vi "medidorIXV.vi"() -> (2 "Corrente Atual":dbl, 3 "Tensao Atual":dbl)   [LabVIEW 2012]
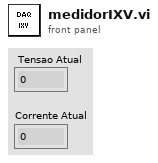
[diagram p1: front panel]
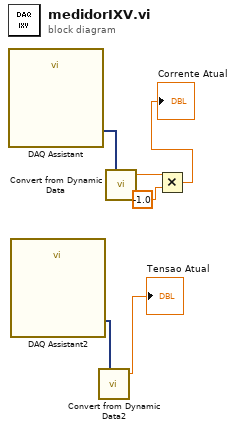
[diagram p0: block diagram]
diagram:
  n1 = call "DAQ Assistant"() -> ("data"=w3:dynamicdata)  [unwired: 17 in, 2 out]
  n2 = call "DAQ Assistant2"() -> ("data"=w1:dynamicdata)  [unwired: 17 in, 2 out]
  n3 = call "Convert from Dynamic Data2"("Dynamic Data Type"=w1) -> ("Scalar"=→"Tensao Atual":dbl)  [unwired: 3 in]
  n4 = call "Convert from Dynamic Data"("Dynamic Data Type"=w3) -> ("Scalar"=w5:dbl)  [unwired: 3 in]
  n5 = Multiply(x=w5, y=-1.0) -> (x*y=→"Corrente Atual":dbl)
